vi "5_3.vi"() -> ()   [LabVIEW 2018]
uses:
  <vilib>/ptbypt/NI_PtbyPt.lvlib
  <vilib>/gmath/NI_Gmath.lvlib
panel:
  in  "观测次数m":dbl
  out "理论误码率":dbl
  out "噪声标准差":dbl
  out "设计误码率":ext
  out "理论最优门限":dbl
  out "先验概率P(H1)":dbl
  in  "先验概率P(H0)":dbl=0.5
  in  "噪声方差":dbl=0.5
  in  "样本数":u64=1000000
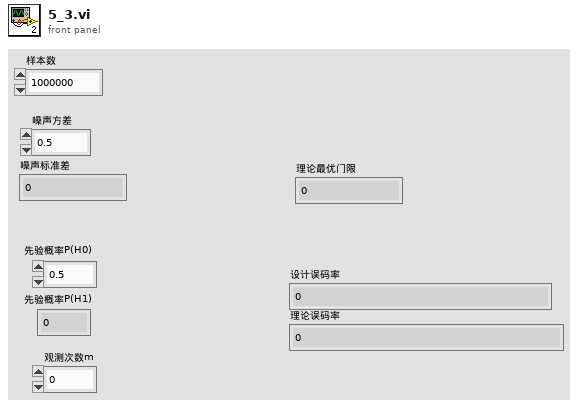
[diagram p1: front panel]
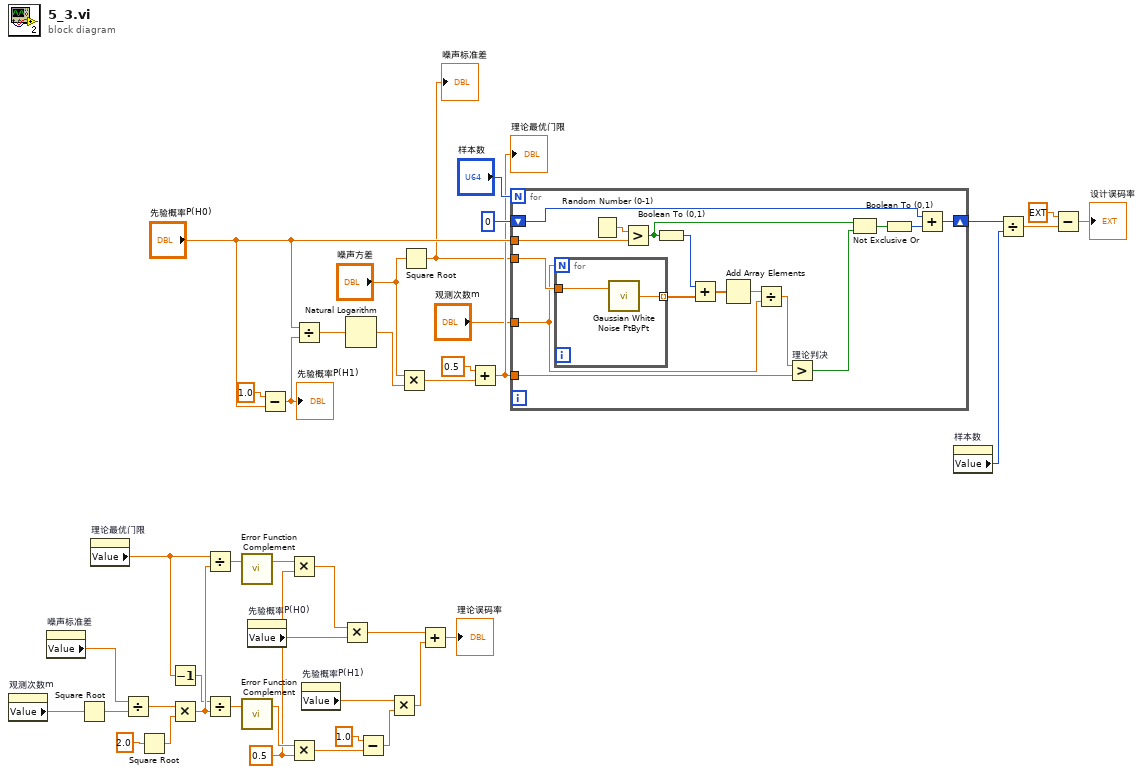
[diagram p0: block diagram]
diagram:
  w21 = 0.5 ("y")
  n1 = property on="观测次数m" class="DigNum (严格)"() -> ("Value"=w6:dbl)  [unwired: 2 in, 2 out]
  n2 = property on="噪声标准差" class="DigNum (严格)"() -> ("Value"=w5:dbl)  [unwired: 2 in, 2 out]
  n3 = Square Root(x=w6) -> (sqrt(x)=w4:dbl)
  n4 = property on="理论最优门限" class="DigNum (严格)"() -> ("Value"=w27:dbl)  [unwired: 2 in, 2 out]
  n5 = Divide(x=w5, y=w4) -> (x/y=w3:dbl)
  n6 = Square Root(x=2.0) -> (sqrt(x)=w29:dbl)
  n7 = Decrement(x=w27) -> (x-1=w26:dbl)
  n8 = Multiply(x=w3, y=w29) -> (x*y=w28:dbl)
  n9 = Divide(x=w27, y=w28) -> (x/y=w25:dbl)
  n10 = Divide(x=w26, y=w28) -> (x/y=w24:dbl)
  n11 = call <vilib>:"Error Function Complement.vi"("x"=w25) -> ("1 - erf(x)"=w22:dbl)  [unwired: 2 in]
  n12 = call <vilib>:"Error Function Complement.vi"("x"=w24) -> ("1 - erf(x)"=w23:dbl)  [unwired: 2 in]
  n13 = property on="先验概率P(H0)" class="DigNum (严格)"() -> ("Value"=w13:dbl)  [unwired: 2 in, 2 out]
  n14 = Subtract(x=1.0, y="先验概率P(H0)") -> (x-y=w33:dbl)
  "先验概率P(H1)" <- w33
  n15 = Multiply(x=w22, y=w21) -> (x*y=w14:dbl)
  n16 = Multiply(x=w23, y=w21) -> (x*y=w20:dbl)
  n17 = Divide(x="先验概率P(H0)", y=w33) -> (x/y=w39:dbl)
  n18 = property on="先验概率P(H1)" class="DigNum (严格)"() -> ("Value"=w12:dbl)  [unwired: 2 in, 2 out]
  n19 = Multiply(x=w14, y=w13) -> (x*y=w9:dbl)
  n20 = Natural Logarithm(1:w39) -> (0:w38:dbl)
  n21 = Subtract(x=1.0, y=w20) -> (x-y=w11:dbl)
  n22 = Multiply(x=w12, y=w11) -> (x*y=w10:dbl)
  n23 = Multiply(x="噪声方差", y=w38) -> (x*y=w37:dbl)
  n24 = Square Root(x="噪声方差") -> (sqrt(x)=w7:dbl)
  "噪声标准差" <- w7
  n25 = Add(x=w9, y=w10) -> (x+y=→"理论误码率":dbl)
  n26 = Add(x=0.5, y=w37) -> (x+y=w31:dbl)
  "理论最优门限" <- w31
  n27 = for {
    N: "样本数" -> [_]
    tunnel: "先验概率P(H0)" -> [w56]
    tunnel: w31 -> [w55]
    shift-right: [w53] -> w2
    shift-left: u64 0 ("元素") -> [w51]
    tunnel: "观测次数m" -> [w43]
    tunnel: w7 -> [w47]
    n28 = for {
      N: w43 -> [_]
      tunnel: w47 -> [w59]
      tunnel: [w58] -> w46 mode=indexing
      n29 = call <vilib>:"Gaussian White Noise PtByPt.vi"("standard deviation"=w59) -> ("Gaussian white noise"=w58:dbl)  [unwired: 2 in]
    }
    n30 = Random Number (0-1)() -> (number: 0 to 1=w57:dbl)
    n31 = Greater?(x=w57, y=w56) -> (0:w48:bool)
    n32 = Boolean To (0,1)(Boolean=w48) -> (0, 1=w50:i16)
    n33 = Add(x=w50, y=w46) -> (x+y=w45:dbl[])
    n34 = Add Array Elements(numeric array=w45) -> (sum=w44:dbl)
    n35 = Divide(x=w44, y=w43) -> (x/y=w42:dbl)
    n36 = Greater? "理论判决"(x=w42, y=w55) -> (0:w54:bool)
    n37 = Not Exclusive Or(1:w54, 2:w48) -> (0:w49:bool)
    n38 = Boolean To (0,1)(Boolean=w49) -> (0, 1=w52:i16)
    n39 = Add(x=w51, y=w52) -> (x+y=w53:u64)
  }
  n40 = property on="样本数" class="DigNum (严格)"() -> ("Value"=w1:u64)  [unwired: 2 in, 2 out]
  n41 = Divide(x=w2, y=w1) -> (x/y=w17:dbl)
  n42 = Subtract(x=ext 1.0, y=w17) -> (x-y=→"设计误码率":ext)
